vi "TS.GetSocketByThread.vi"(8 "error in":errorcluster, 11 "TS.Thread ref in":refnum<k7>) -> (0 "error out":errorcluster, 2 "socket":dbl)   [LabVIEW 2019, in "Tools.lvlib"]
uses:
  Tools.lvlib
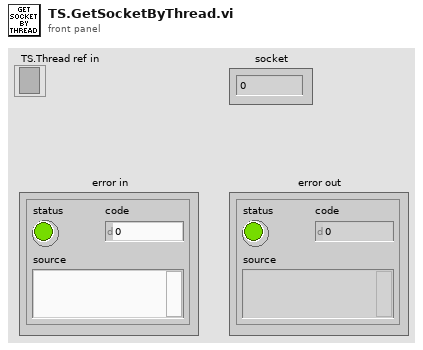
[diagram p1: front panel]
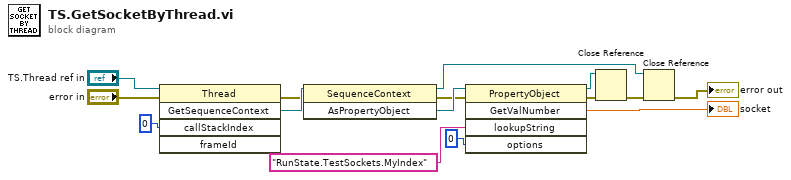
[diagram p0: block diagram]
diagram:
  n1 = invoke class="Thread" method="GetSequenceContext"(reference="TS.Thread ref in", error in="error in", "callStackIndex"=0) -> (error out=w8:errorcluster, "GetSequenceContext"=w13:refnum<k7>)  [unwired: 2 in, 3 out]
  n2 = invoke class="SequenceContext" method="AsPropertyObject"(reference=w13, error in=w8) -> (reference out=w1:refnum<k7>, error out=w7:errorcluster, "AsPropertyObject"=w12:refnum<k7>)  [unwired: 1 in]
  n3 = invoke class="PropertyObject" method="GetValNumber"(reference=w12, error in=w7, "lookupString"="RunState.TestSockets.MyIndex", "options"=0) -> (reference out=w6:refnum<k7>, error out=w5:errorcluster, "GetValNumber"=→"socket":dbl)  [unwired: 1 in, 2 out]
  n4 = Close Reference(reference=w6, error in (no error)=w5) -> (error out=w4:errorcluster)
  n5 = Close Reference(reference=w1, error in (no error)=w4) -> (error out=→"error out":errorcluster)
